vi "Coding Constant.vi"() -> (2 "Constant out":T1)   [LabVIEW 2017]
uses:
  Default volues.vi
panel:
  in  "Coding Constant":T1={"Th_A"=0.05, "Th_B"=0.5, "Th_C"=2.0, "ChupLimt"=0.9, "ChdnLimt"=0.1, "Bcd"=0, "StepMem"=0} {"Bcd" format="%b"}
  # "修改初始值，需要置当前值为缺省值，然后保存VI。"
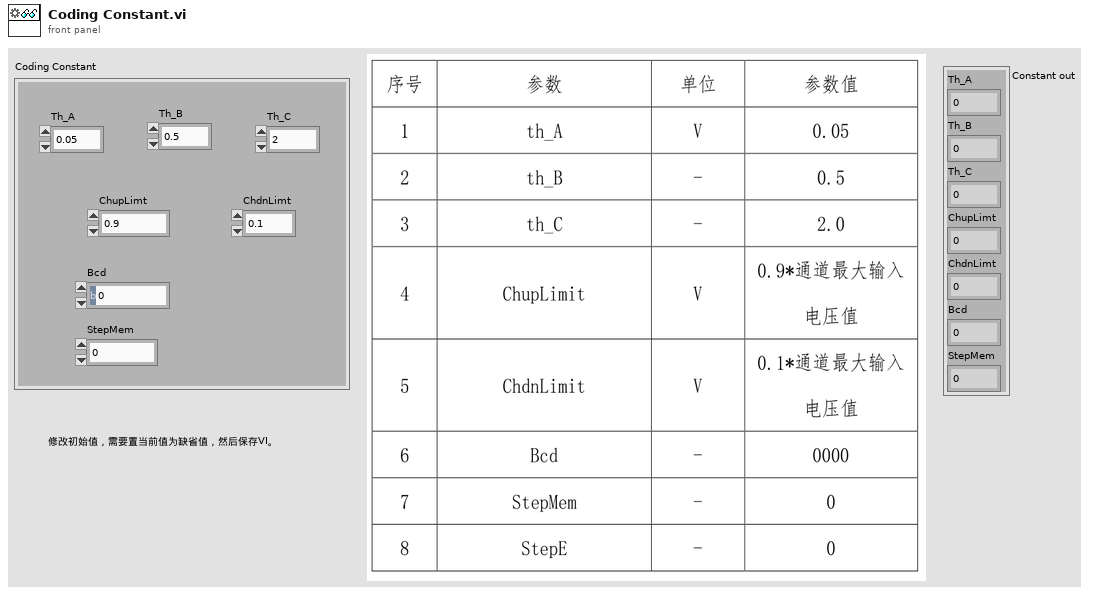
[diagram p1: front panel]
types:
  T1 = cluster{"Th_A":dbl, "Th_B":dbl, "Th_C":dbl, "ChupLimt":dbl, "ChdnLimt":dbl, "Bcd":u8, "StepMem":u32}
  T2 = cluster{"AI Channel":tag, "Min Voltage":dbl, "Max Voltage":dbl, "Terminal Configuration":i32, "Sample Rate":dbl, "Number of Samples":i32, "Logging Mode":i32, "TDMS File Path":path, "Digital Start Trigger Source":tag, "Digital Start Trigger Edge":i32}
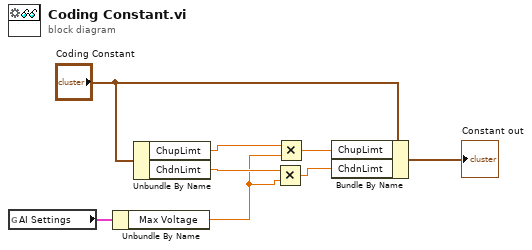
[diagram p0: block diagram]
diagram:
  n1 = global read "Default volues.vi" "AI Settings"() -> (w8:T2)
  n2 = Unbundle By Name(w8) -> ("Max Voltage"=w2:dbl)
  n3 = Unbundle By Name("Coding Constant") -> ("ChupLimt"=w5:dbl, "ChdnLimt"=w4:dbl)
  n4 = Multiply(x=w4, y=w2) -> (x*y=w3:dbl)
  n5 = Multiply(x=w5, y=w2) -> (x*y=w6:dbl)
  n6 = Bundle By Name(cluster="Coding Constant", "ChupLimt"=w6, "ChdnLimt"=w3) -> (→"Constant out":T1)
